vi "Index Arrays - string.vi"(9 "Index array":u32[](array[numeric]), 11 "Array in":string[](array[string])) -> (3 "Array out":string[](array[string]))   [LabVIEW 2014]
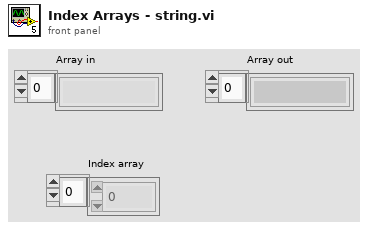
[diagram p1: front panel]
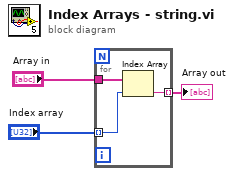
[diagram p0: block diagram]
diagram:
  n1 = for {
    tunnel: "Index array" -> [w6] mode=indexing
    tunnel: [w5] -> w1 mode=indexing
    tunnel: "Array in" -> [w4]
    n2 = Index Array(array=w4, index=w6) -> (element=w5:string)
  }
  "Array out" <- w1
